vi "Receive Value Change Event.vi"(8 "error in (no error)":errorcluster, 10 "ValueChangeMsg":refnum<class "ValueChangeMsg.lvclass">, 11 "For Loop Dialog In":refnum<class "Sequence Dialog.lvclass">) -> (0 "error out":errorcluster, 3 "For Loop Dialog Out":refnum<class "Sequence Dialog.lvclass">)   [LabVIEW 2020, in "Sequence Dialog.lvclass"]
doc: "<License>\nCopyright © 2017 Composed Systems, LLC | All rights reserved\nwww.composed.io\n\nAuthor: Ethan Stern <ethan.stern@composed.io>\n\nThis software is provided \"AS IS\" WITHOUT WARRANTIES, either express or implied, AND IS FOR EDUCATIONAL PURPOSES ONLY.\n</License>"
uses:
  <vilib>/gpm_packages/@cs/Test-executive-builder/Source/Test Executive Builder Dialogs/Edit Sequence Dialog/Sequence Dialog.lvclass
  C:/Program Files/National Instruments/LabVIEW 2020/vi.lib/ActorFramework/Actor/Actor.lvclass
  C:/Program Files/National Instruments/LabVIEW 2020/vi.lib/gpm_packages/@cs/Test-executive-builder/Source/Test Executive Builder Dialogs/ITest Executive Builder Dialog/ITest Executive Builder Dialog.lvclass
  C:/Program Files/National Instruments/LabVIEW 2020/vi.lib/gpm_packages/@cs/popup-viewmanager/Source/Popup ViewManager/Popup ViewManager.lvclass
  <vilib>/gpm_packages/@cs/mva-viewable/Source/ActorEvents/IEventAggregator Messages/ValueChangeMsg/ValueChangeMsg.lvclass
  <vilib>/gpm_packages/@cs/mva-viewable/Source/ActorEvents/IEventAggregator Messages/ValueChangeMsg/ValueChangeMsg.lvclass/ValueChangeMsg.ctl
  <vilib>/ActorFramework/Actor/Actor.lvclass/Actor.ctl
  <vilib>/ActorFramework/Message Enqueuer/Message Enqueuer.lvclass/Message Enqueuer.ctl
  <vilib>/gpm_packages/@cs/Test-executive-builder/Source/Test Executive Builder Dialogs/Edit Sequence Dialog/Sequence Dialog.lvclass/Sequence Dialog.ctl
  <vilib>/gpm_packages/@cs/Test-executive-builder/Source/Test Executive Builder Dialogs/ITest Executive Builder Dialog/ITest Executive Builder Dialog.lvclass/ITest Executive Builder Dialog.ctl
  <vilib>/gpm_packages/@cs/mva-viewable/Source/IViewable/IViewable Messages/Insert Front Panel Msg/Insert Front Panel Msg.lvclass/Insert Front Panel Msg.ctl
  <vilib>/gpm_packages/@cs/Test-executive-builder/Source/Test Executive Builder Dialogs/IAttribute Data Type View Messages/Set Value Msg/Set Value Msg.lvclass/Set Value Msg.ctl
  <vilib>/ActorFramework/Message Enqueuer/Init from Existing Queue.vi
  <vilib>/ActorFramework/Message Enqueuer/Enqueue.vi
  <vilib>/ActorFramework/Stop Msg/Stop Msg.lvclass
  C:/Program Files/National Instruments/LabVIEW 2020/vi.lib/ActorFramework/Message/Message.lvclass
  <vilib>/gpm_packages/@cs/mva-viewable/Source/IViewable/IViewable Messages/Insert Front Panel Msg/Insert Front Panel Msg.lvclass
  <vilib>/gpm_packages/@cs/Test-executive-builder/Source/Test Executive Builder Dialogs/IAttribute Data Type View Messages/Set Value Msg/Set Value Msg.lvclass
  <vilib>/ActorFramework/Message Priority Queue/Priority Enqueue.vi
  <vilib>/ActorFramework/Message Enqueuer/Message Enqueuer.lvclass
  <vilib>/gpm_packages/@cs/Test-executive-builder/Source/Test Executive Builder Dialogs/ITest Executive Builder Dialog/ITest Executive Builder Dialog.lvclass
  <vilib>/gpm_packages/@cs/Test-executive-builder/Source/Data Type Handler/Test Executive Builder Data Type Handler.lvclass
  <vilib>/ActorFramework/Actor/Actor.lvclass
  <vilib>/gpm_packages/@cs/popup-viewmanager/Source/Popup ViewManager/Popup ViewManager.lvclass
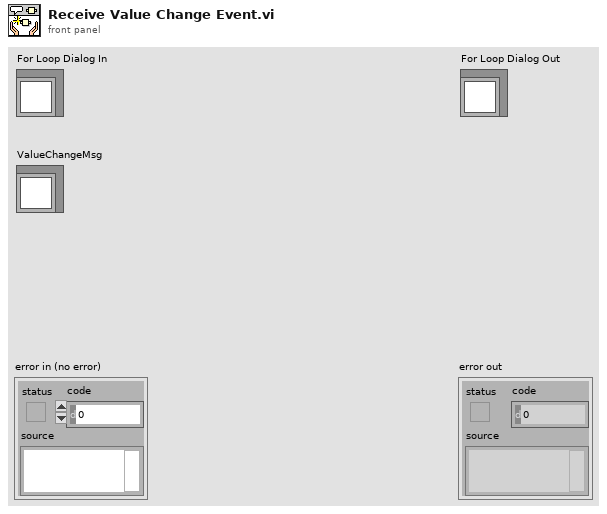
[diagram p1: front panel]
types:
  T1 = typedef "IViewable.lvlib/ProtectedSubpanel.lvclass/Protected Subpanel Reference.ctl" = refnum<data-value>
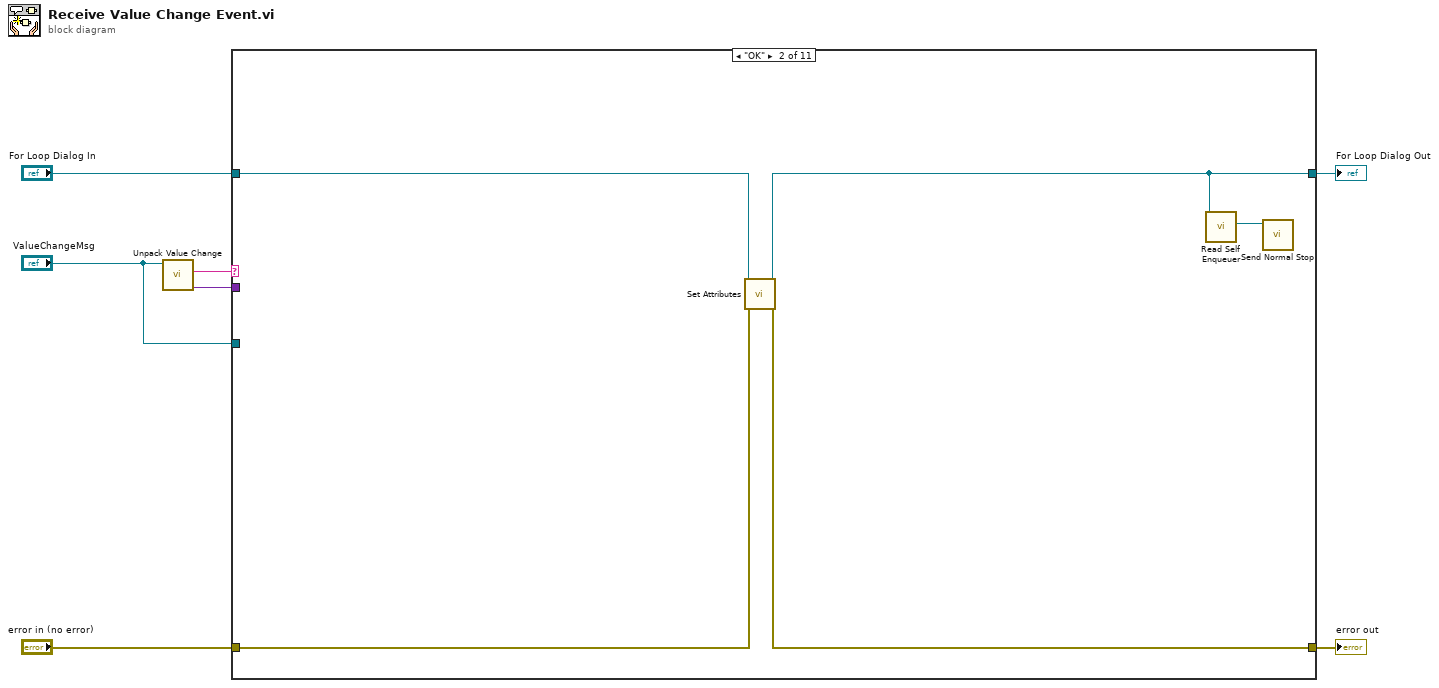
[diagram p0: block diagram]
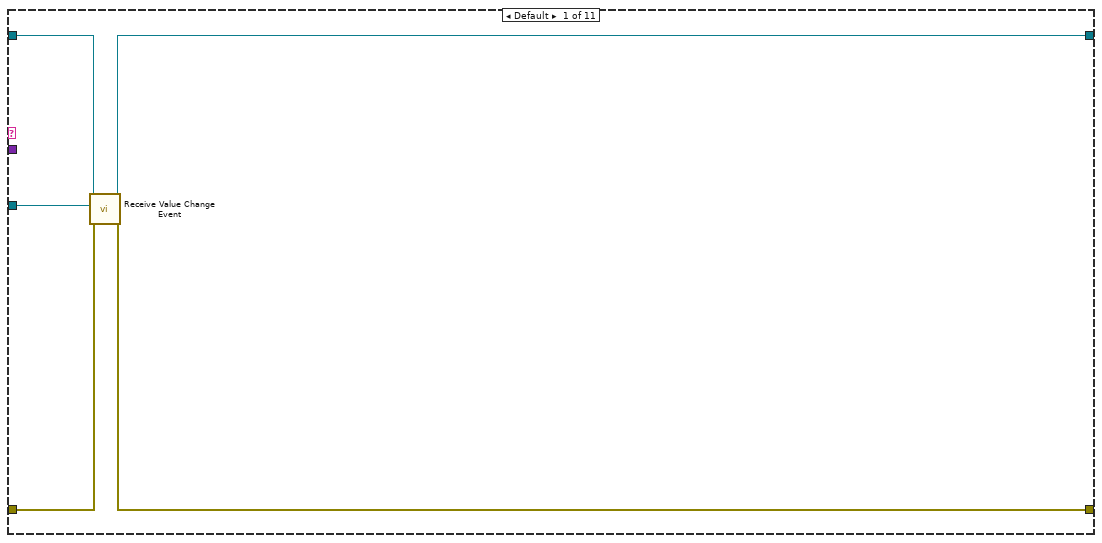
[diagram p2: hidden frame]
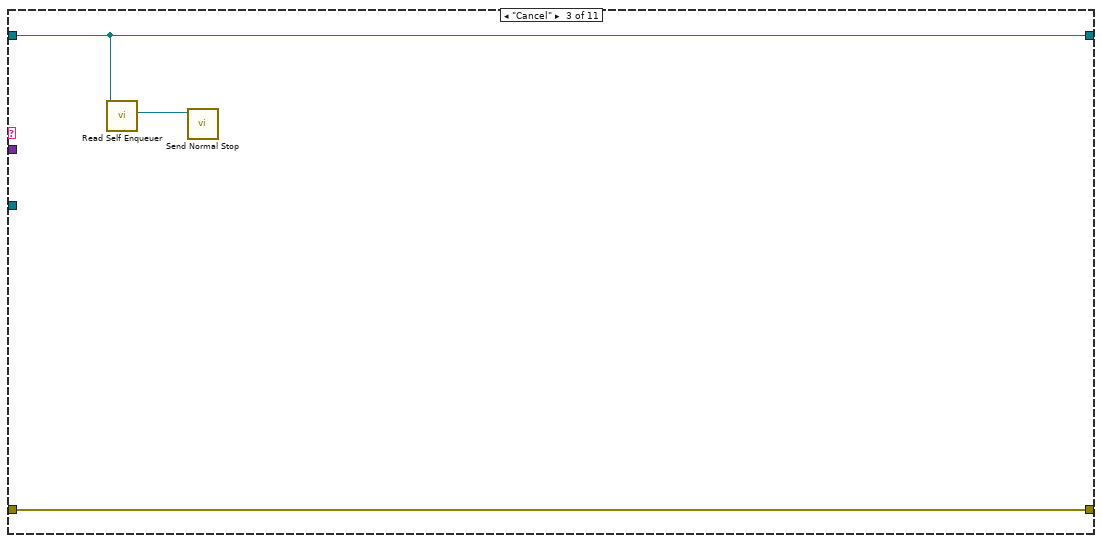
[diagram p3: hidden frame]
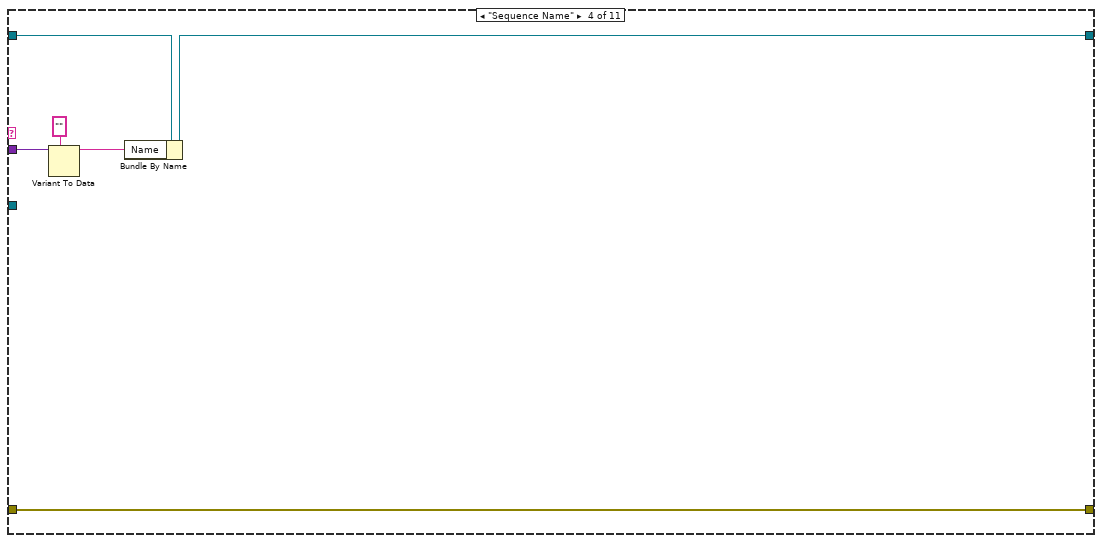
[diagram p4: hidden frame]
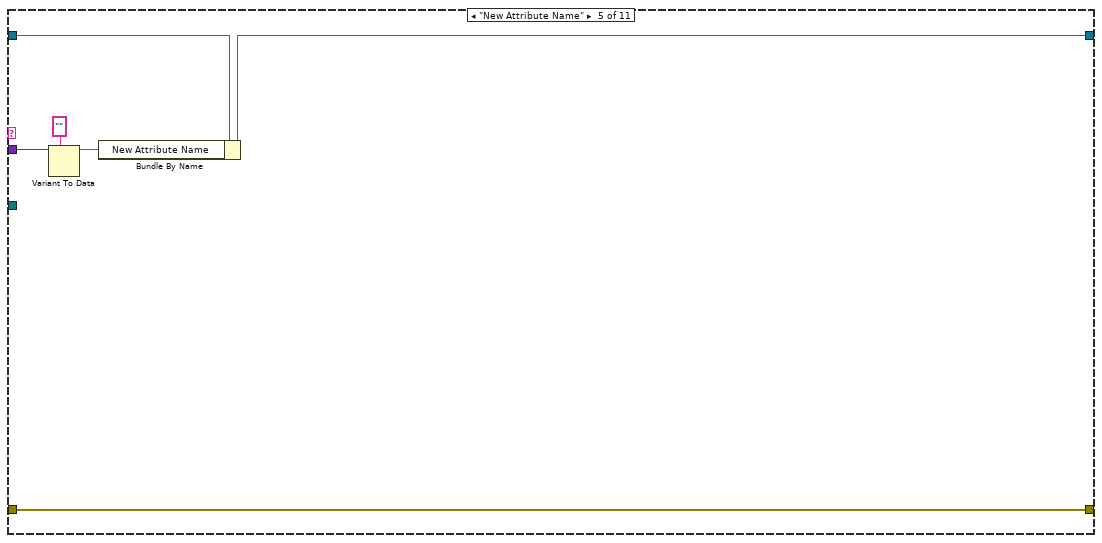
[diagram p5: hidden frame]
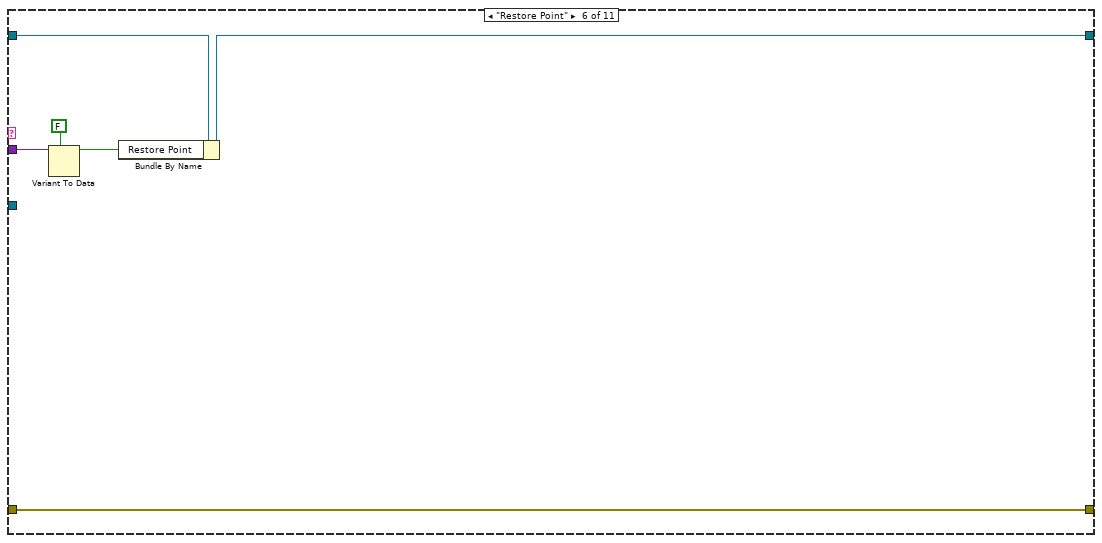
[diagram p6: hidden frame]
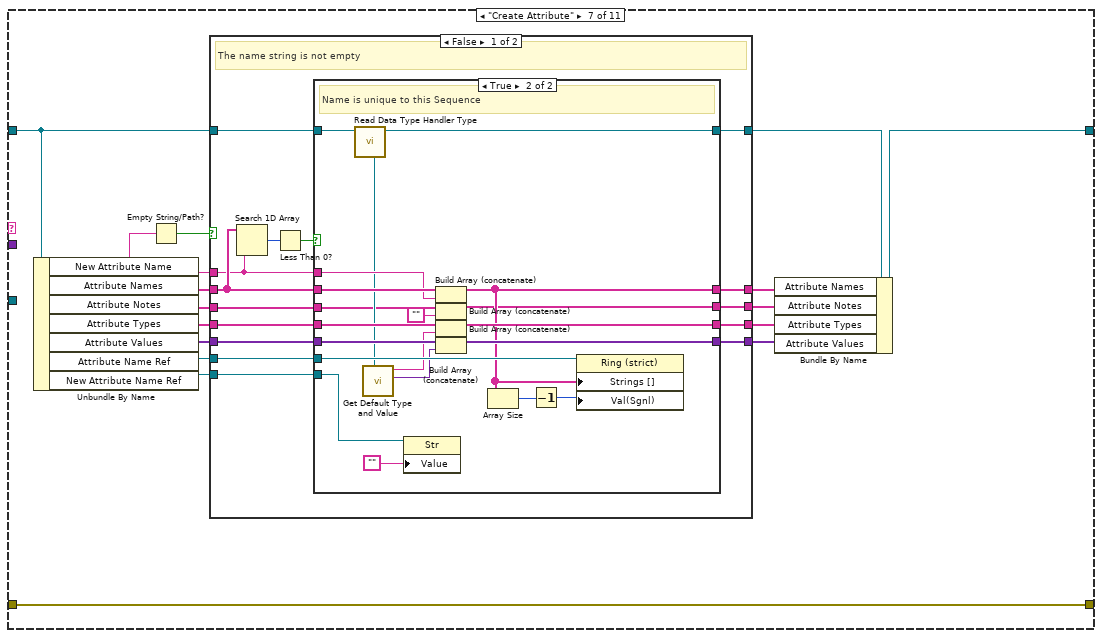
[diagram p7: hidden frame]
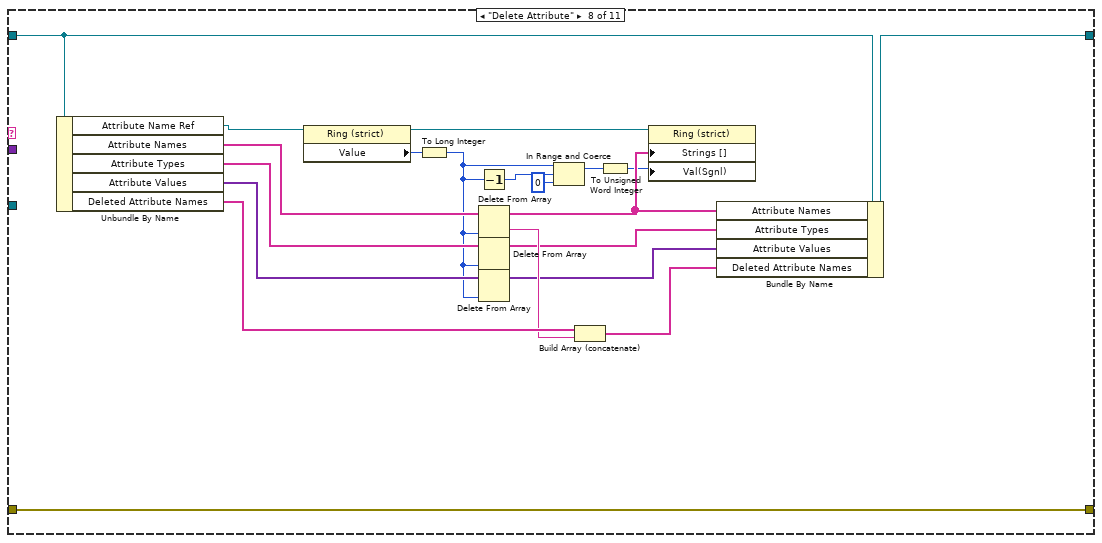
[diagram p10: hidden frame]
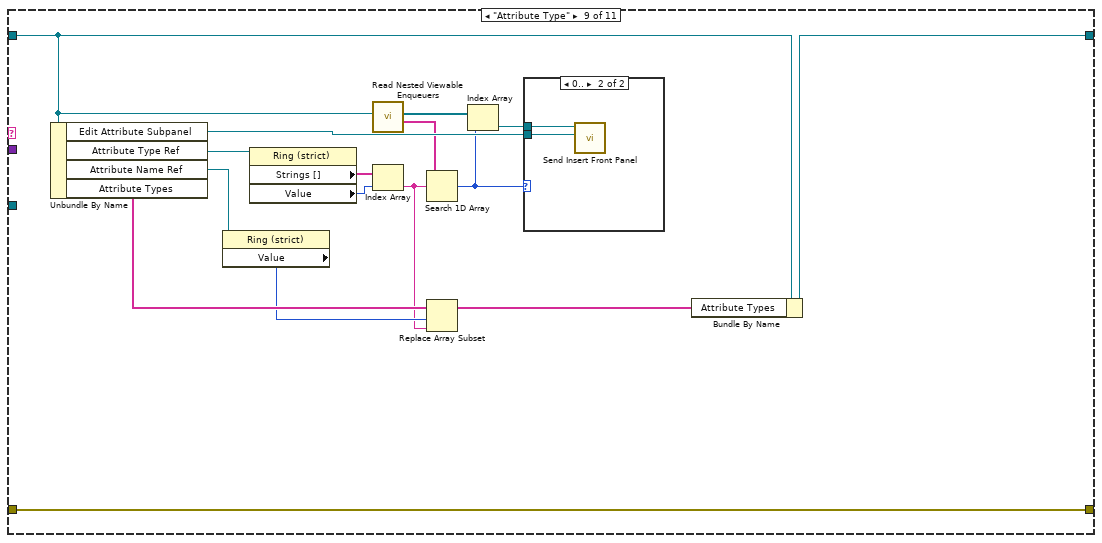
[diagram p11: hidden frame]
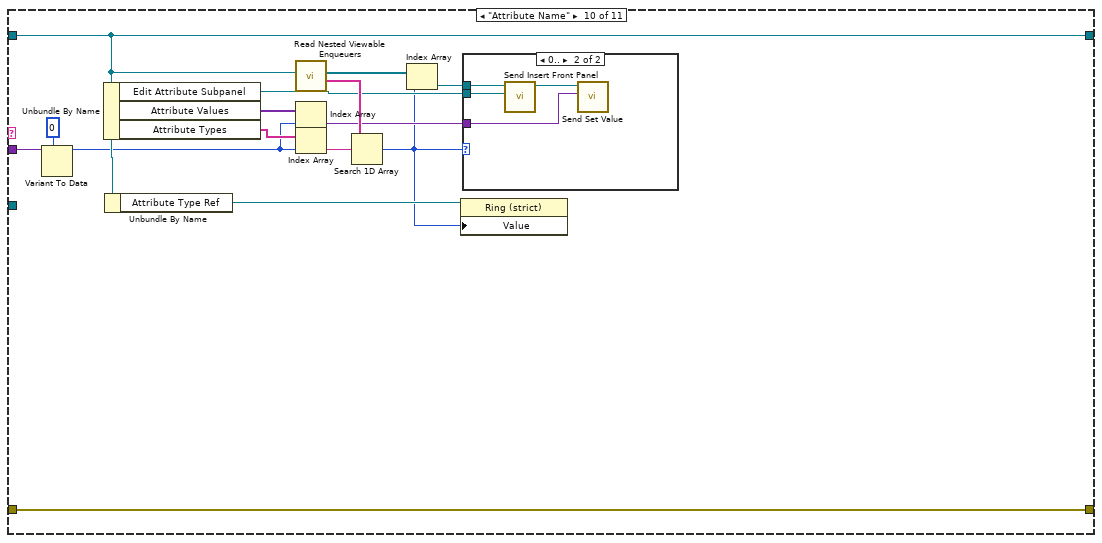
[diagram p13: hidden frame]
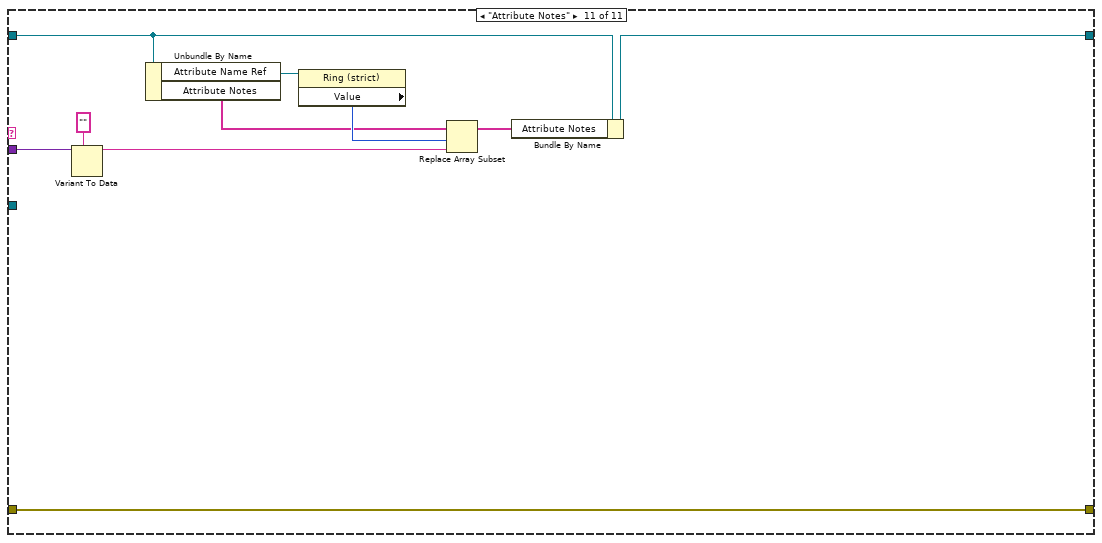
[diagram p15: hidden frame]
diagram:
  n1 = call <vilib>:"Unpack Value Change.vi"("ValueChangeMsg"="ValueChangeMsg") -> ("New Value"=w1:variant, "Control Label"=w2:string)  [unwired: 6 in, 3 out]
  n2 = case shown="\"OK\"" w2 {
    tunnel: [w12 w13 w20 w26 w32 w38 w54 w119 w135 w152 w166] -> w7
    tunnel: [w11 w15 w19 w21 w27 w33 w45 w109 w121 w141 w158] -> w6
    tunnel: "error in (no error)" -> [w10 w14 w20 w26 w32 w38 w54 w119 w135 w152 w166]
    tunnel: "For Loop Dialog In" -> [w9 w16 w19 w22 w28 w34 w47 w110 w122 w141 w159]
    tunnel: "ValueChangeMsg" -> [w8 _ _ _ _ _ _ _ _ _ _]
    tunnel: w1 -> [_ _ _ w25 w31 w37 _ _ _ w151 w162]
    frame Default {
      n3 = call-parent "Receive Value Change Event.vi"("error in (no error)"=w10, "ValueChangeMsg"=w8, "IViewable In"=w9) -> ("error out"=w12:errorcluster, "IViewable Out"=w11:refnum<class "Sequence Dialog.lvclass">)  [unwired: 7 in]
    }
    frame "OK" {
      n4 = call-dynamic "Set Attributes.vi"("error in (no error)"=w14, "Sequence Dialog in"=w16) -> ("error out"=w13:errorcluster, "Sequence Dialog out"=w15:refnum<class "Sequence Dialog.lvclass">)  [unwired: 8 in]
      n5 = call <vilib>:"Read Self Enqueuer.vi"("Actor"=w15) -> ("Self Enqueuer"=w17:refnum<class "Message Enqueuer.lvclass">)  [unwired: 10 in]
      n6 = call <vilib>:"Send Normal Stop.vi"("Message Enqueuer"=w17) -> ()  [unwired: 10 in, 1 out]
    }
    frame "Cancel" {
      n7 = call <vilib>:"Read Self Enqueuer.vi"("Actor"=w19) -> ("Self Enqueuer"=w18:refnum<class "Message Enqueuer.lvclass">)  [unwired: 10 in]
      n8 = call <vilib>:"Send Normal Stop.vi"("Message Enqueuer"=w18) -> ()  [unwired: 10 in, 1 out]
    }
    frame "Sequence Name" {
      n9 = Variant To Data(type="" ("Iterations"), Variant=w25) -> (data=w23:string)  [unwired: 1 in, 1 out]
      n10 = Bundle By Name(cluster=w22, "Name"=w23) -> (w21:refnum<class "Sequence Dialog.lvclass">)
    }
    frame "New Attribute Name" {
      n11 = Variant To Data(type="" ("Iterations"), Variant=w31) -> (data=w29:string)  [unwired: 1 in, 1 out]
      n12 = Bundle By Name(cluster=w28, "New Attribute Name"=w29) -> (w27:refnum<class "Sequence Dialog.lvclass">)
    }
    frame "Restore Point" {
      n13 = Variant To Data(type=FALSE, Variant=w37) -> (data=w35:bool)  [unwired: 1 in, 1 out]
      n14 = Bundle By Name(cluster=w34, "Restore Point"=w35) -> (w33:refnum<class "Sequence Dialog.lvclass">)
    }
    frame "Create Attribute" {
      n15 = Unbundle By Name(w47) -> ("New Attribute Name"=w53:string, "Attribute Names"=w51:string[], "Attribute Notes"=w41:string[], "Attribute Types"=w50:string[], "Attribute Values"=w49:variant[], "Attribute Name Ref"=w48:refnum<vi>, "New Attribute Name Ref"=w39:refnum<vi>)
      n16 = Empty String/Path?(string/path=w53) -> (empty?=w52:bool)
      n17 = case shown="False" w52 {
        tunnel: w53 -> [w63 _]
        tunnel: w51 -> [w67 w99]
        tunnel: w50 -> [w66 w98]
        tunnel: w49 -> [w65 w97]
        tunnel: w48 -> [w64 _]
        tunnel: [w62 w99] -> w44
        tunnel: [w61 w98] -> w43
        tunnel: [w60 w97] -> w42
        tunnel: [w59 w96] -> w46
        tunnel: w47 -> [w58 w96]
        tunnel: w41 -> [w57 w95]
        tunnel: [w56 w95] -> w40
        tunnel: w39 -> [w55 _]
        frame False {
          # "The name string is not empty"
          n18 = Search 1D Array(1D array=w67, element=w63) -> (index of element=w68:i32)  [unwired: 1 in]
          n19 = Less Than 0?(x=w68) -> (x < 0?=w69:bool)
          n20 = case shown="True" w69 {
            tunnel: w67 -> [w74 w94]
            tunnel: w66 -> [w73 w92]
            tunnel: w65 -> [w72 w91]
            tunnel: w64 -> [_ w87]
            tunnel: w63 -> [_ w93]
            tunnel: [w74 w86] -> w62
            tunnel: [w73 w90] -> w61
            tunnel: [w72 w89] -> w60
            tunnel: [w71 w83] -> w59
            tunnel: w58 -> [w71 w84]
            tunnel: w57 -> [w70 w79]
            tunnel: [w70 w77] -> w56
            tunnel: w55 -> [_ w75]
            frame False {
              # "Name is not unique"
            }
            frame True {
              # "Name is unique to this Sequence"
              n21 = call <vilib>:"Read Data Type Handler Type.vi"("ITest Executive Builder Dialog in"=w84) -> ("ITest Executive Builder Dialog out"=w83:refnum<class "Sequence Dialog.lvclass">, "Data Type Handler"=w82:refnum<class "Test Executive Builder Data Type Handler.lvclass">)  [unwired: 9 in]
              n22 = call-dynamic "Get Default Type and Value.vi"("Test Executive Builder Data Type Handler in"=w82) -> ("Default Value"=w80:variant, "Default Type"=w81:string)  [unwired: 9 in]
              n23 = property class="Str"(reference=w75, "Value"="") -> ()  [unwired: 1 in, 2 out]
              n24 = Build Array (concatenate)(w94, w93) -> (w86:string[])
              n25 = Build Array (concatenate)(w79, "") -> (w77:string[])
              n26 = Build Array (concatenate)(w92, w81) -> (w90:string[])
              n27 = Build Array (concatenate)(w91, w80) -> (w89:variant[])
              n28 = Array Size(array=w86) -> (size(s)=w88:i32)
              n29 = Decrement(x=w88) -> (x-1=w85:i32)
              n30 = property class="Ring (strict)"(reference=w87, "Strings []"=w86, "Val(Sgnl)"=w85) -> ()  [unwired: 1 in, 2 out]
            }
          }
        }
        frame True {
          # "The new attribute must have a name"
        }
      }
      n31 = Bundle By Name(cluster=w46, "Attribute Names"=w44, "Attribute Notes"=w40, "Attribute Types"=w43, "Attribute Values"=w42) -> (w45:refnum<class "Sequence Dialog.lvclass">)
    }
    frame "Delete Attribute" {
      n32 = Unbundle By Name(w110) -> ("Attribute Name Ref"=w118:refnum<vi>, "Attribute Names"=w117:string[], "Attribute Types"=w115:string[], "Attribute Values"=w114:variant[], "Deleted Attribute Names"=w113:string[])
      n33 = property class="Ring (strict)"(reference=w118) -> (reference out=w111:refnum<vi>, "Value"=w116:u16)  [unwired: 1 in, 1 out]
      n34 = To Long Integer(number=w116) -> (32bit integer=w104:i32)
      n35 = Decrement(x=w104) -> (x-1=w103:i32)
      n36 = Delete From Array(array=w117, index=w104) -> (deleted portion=w112:string, array with subset deleted=w108:string[])  [unwired: 1 in]
      n37 = Delete From Array(array=w115, index=w104) -> (array with subset deleted=w107:string[])  [unwired: 1 in, 1 out]
      n38 = Delete From Array(array=w114, index=w104) -> (array with subset deleted=w106:variant[])  [unwired: 1 in, 1 out]
      n39 = In Range and Coerce(upper limit=w104, x=w103, lower limit=0) -> (coerced(x)=w101:i32)  [unwired: 1 out]
      n40 = Build Array (concatenate)(w113, w112) -> (w105:string[])
      n41 = To Unsigned Word Integer(number=w101) -> (unsigned 16bit integer=w100:u16)
      n42 = property class="Ring (strict)"(reference=w111, "Strings []"=w108, "Val(Sgnl)"=w100) -> ()  [unwired: 1 in, 2 out]
      n43 = Bundle By Name(cluster=w110, "Attribute Names"=w108, "Attribute Types"=w107, "Attribute Values"=w106, "Deleted Attribute Names"=w105) -> (w109:refnum<class "Sequence Dialog.lvclass">)
    }
    frame "Attribute Type" {
      n44 = Unbundle By Name(w122) -> ("Edit Attribute Subpanel"=w131:T1, "Attribute Type Ref"=w134:refnum<vi>, "Attribute Name Ref"=w126:refnum<vi>, "Attribute Types"=w125:string[])
      n45 = property class="Ring (strict)"(reference=w126) -> ("Value"=w124:u16)  [unwired: 1 in, 2 out]
      n46 = property class="Ring (strict)"(reference=w134) -> ("Strings []"=w130:string[], "Value"=w129:u16)  [unwired: 1 in, 2 out]
      n47 = call <vilib>:"Read Nested Viewable Enqueuers.vi"("Popup ViewManager in"=w122) -> ("Viewable Names"=w128:string[], "Nested Enqueuers"=w133:refnum<class "Message Enqueuer.lvclass">[])  [unwired: 9 in]
      n48 = Index Array(array=w130, index=w129) -> (element=w123:string)
      n49 = Search 1D Array(1D array=w128, element=w123) -> (index of element=w127:i32)  [unwired: 1 in]
      n50 = Replace Array Subset(array=w125, new element=w123, index=w124) -> (w120:string[])
      n51 = Index Array(array=w133, index=w127) -> (element=w132:refnum<class "Message Enqueuer.lvclass">)
      n52 = case shown="0.." w127 {
        tunnel: w132 -> [_ w137]
        tunnel: w131 -> [_ w136]
        frame Default {
        }
        frame 0.. {
          n53 = call <vilib>:"Send Insert Front Panel.vi"("Protected Subpanel"=w136, "Message Enqueuer"=w137) -> ()  [unwired: 8 in, 2 out]
        }
      }
      n54 = Bundle By Name(cluster=w122, "Attribute Types"=w120) -> (w121:refnum<class "Sequence Dialog.lvclass">)
    }
    frame "Attribute Name" {
      n55 = Variant To Data(type=u16 0, Variant=w151) -> (data=w139:u16)  [unwired: 1 in, 1 out]
      n56 = Unbundle By Name(w141) -> ("Edit Attribute Subpanel"=w143:T1, "Attribute Values"=w148:variant[], "Attribute Types"=w149:string[])
      n57 = Unbundle By Name(w141) -> ("Attribute Type Ref"=w140:refnum<vi>)
      n58 = call <vilib>:"Read Nested Viewable Enqueuers.vi"("Popup ViewManager in"=w141) -> ("Viewable Names"=w145:string[], "Nested Enqueuers"=w147:refnum<class "Message Enqueuer.lvclass">[])  [unwired: 9 in]
      n59 = Index Array(array=w148, index=w139) -> (element=w142:variant)
      n60 = Index Array(array=w149, index=w139) -> (element=w144:string)
      n61 = Search 1D Array(1D array=w145, element=w144) -> (index of element=w138:i32)  [unwired: 1 in]
      n62 = Index Array(array=w147, index=w138) -> (element=w146:refnum<class "Message Enqueuer.lvclass">)
      n63 = property class="Ring (strict)"(reference=w140, "Value"=w138) -> ()  [unwired: 1 in, 2 out]
      n64 = case shown="0.." w138 {
        tunnel: w146 -> [_ w156]
        tunnel: w143 -> [_ w155]
        tunnel: w142 -> [_ w153]
        frame Default {
        }
        frame 0.. {
          n65 = call <vilib>:"Send Insert Front Panel.vi"("Protected Subpanel"=w155, "Message Enqueuer"=w156) -> ("Message Enqueuer out"=w154:refnum<class "Message Enqueuer.lvclass">)  [unwired: 8 in, 1 out]
          n66 = call <vilib>:"Send Set Value.vi"("Value"=w153, "Message Enqueuer"=w154) -> ()  [unwired: 8 in, 2 out]
        }
      }
    }
    frame "Attribute Notes" {
      n67 = Variant To Data(type="", Variant=w162) -> (data=w160:string)  [unwired: 1 in, 1 out]
      n68 = Unbundle By Name(w159) -> ("Attribute Name Ref"=w165:refnum<vi>, "Attribute Notes"=w163:string[])
      n69 = property class="Ring (strict)"(reference=w165) -> ("Value"=w164:u16)  [unwired: 1 in, 2 out]
      n70 = Replace Array Subset(array=w163, new element=w160, index=w164) -> (w157:string[])
      n71 = Bundle By Name(cluster=w159, "Attribute Notes"=w157) -> (w158:refnum<class "Sequence Dialog.lvclass">)
    }
  }
  "error out" <- w7
  "For Loop Dialog Out" <- w6
